vi "Search Subscriptions for Match.vi"(10 "Subscription":T1, 11 "MVC Subscription in":refnum<class "MVC Subscription.lvclass">) -> (1 "Index":i32, 2 "Found":bool, 3 "MVC Subscription out":refnum<class "MVC Subscription.lvclass">)   [LabVIEW 2014, in "MVC Subscription.lvlib" / "MVC Subscription.lvclass"]
uses:
  MVC Subscription.lvclass
  Cluster - Individual Subscription.ctl
  <vilib>/ActorFramework/Message Enqueuer/Message Enqueuer.lvclass
  <vilib>/ActorFramework/Message/Message.lvclass
  MVC Subscription.lvclass/MVC Subscription.ctl
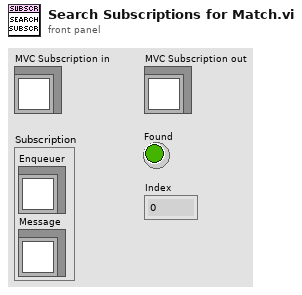
[diagram p1: front panel]
types:
  T1 = typedef "MVC Subscription.lvlib/MVC Subscription.lvclass/Cluster - Individual Subscription.ctl" = cluster{"Enqueuer":refnum<class "Message Enqueuer.lvclass">, "Message":refnum<class "Message.lvclass">}
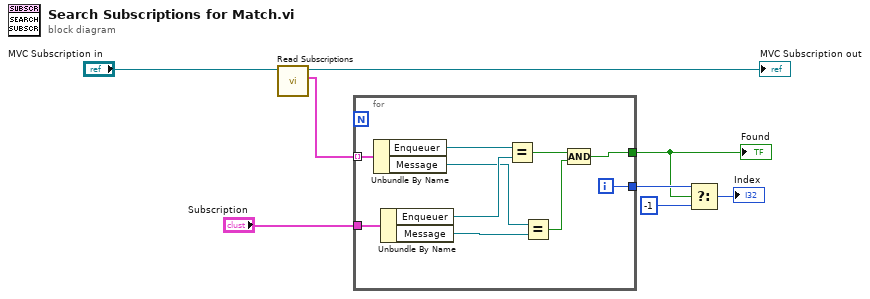
[diagram p0: block diagram]
diagram:
  n1 = call "Read Subscriptions.vi"("MVC Subscription in"="MVC Subscription in") -> ("Subscriptions"=w3:T1[], "MVC Subscription out"=→"MVC Subscription out":refnum<class "MVC Subscription.lvclass">)  [unwired: 9 in]
  n2 = for {
    tunnel: w3 -> [w18] mode=indexing
    tunnel: "Subscription" -> [w17]
    tunnel: [w10] -> w5
    tunnel: [w13] -> w6
    i -> [w13]
    n3 = Unbundle By Name(w18) -> ("Enqueuer"=w16:refnum<class "Message Enqueuer.lvclass">, "Message"=w12:refnum<class "Message.lvclass">)
    n4 = Unbundle By Name(w17) -> ("Enqueuer"=w15:refnum<class "Message Enqueuer.lvclass">, "Message"=w11:refnum<class "Message.lvclass">)
    n5 = Equal?(x=w16, y=w15) -> (x = y?=w14:bool)
    n6 = Equal?(x=w12, y=w11) -> (x = y?=w9:bool)
    n7 = Compound Arithmetic op=AND(w14, w9) -> (w10:bool)
  }
  "Found" <- w5
  n8 = Select(t=w6, s=w5, f=-1) -> (s? t:f=→"Index":i32)
